vi "CreateArrFileName.vi"(4 "BaseDataPath":path, 6 "VarParName":string, 7 "Date":string, 8 "error in (no error)":errorcluster, 9 "PointIndex":i64, 10 "ScanIndex":i64, 11 "SessionInd":i32) -> (0 "error out":errorcluster, 1 "DataFileName":path, 2 "HeadersFileName":path)   [LabVIEW 2019, in "Interface.lvclass"]
doc: "Ce VI sauvegarde les données d'acquisition pour en garder une copie de sécurité qui peut être rappeller en cas de panne."
uses:
  Interface Class/Interface.lvclass
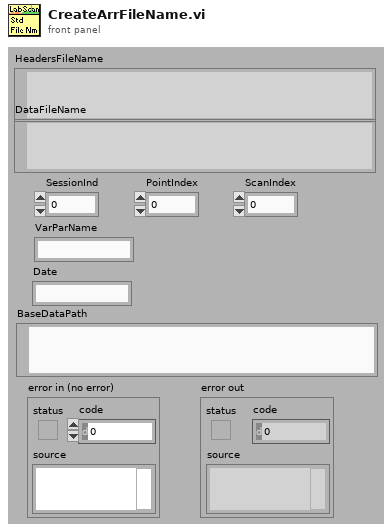
[diagram p1: front panel]
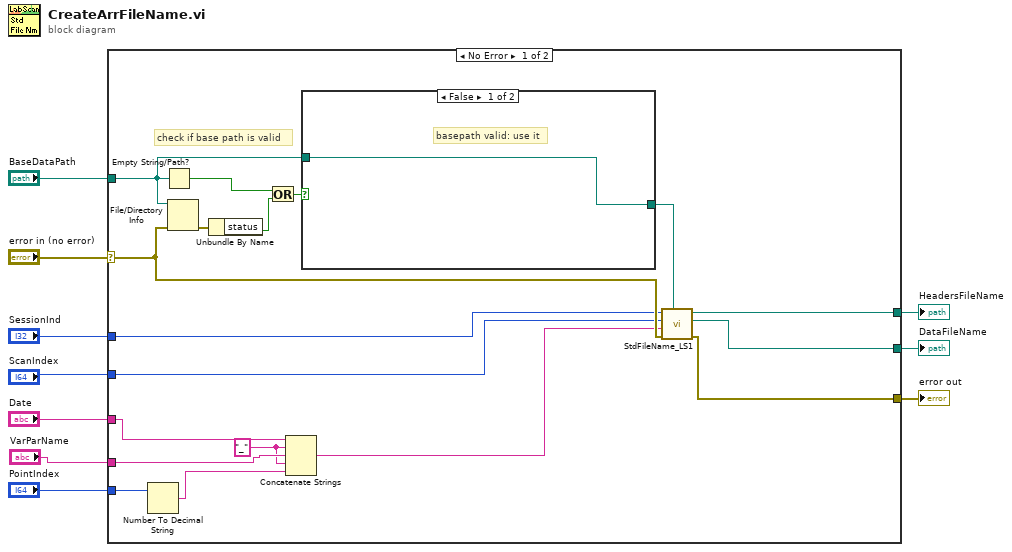
[diagram p0: block diagram]
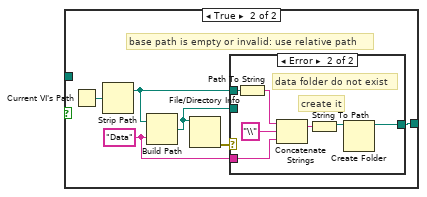
[diagram p2: hidden frame]
diagram:
  n1 = case shown="No Error" "error in (no error)" {
    selector: "error in (no error)" -> [w22 w44]
    tunnel: [w24 w44] -> w9
    tunnel: "Date" -> [w16 _]
    tunnel: [w21 _] -> w7
    tunnel: [w20 _] -> w6
    tunnel: "ScanIndex" -> [w19 _]
    tunnel: "BaseDataPath" -> [w18 _]
    tunnel: "SessionInd" -> [w17 _]
    tunnel: "VarParName" -> [w15 _]
    tunnel: "PointIndex" -> [w13 _]
    frame No Error {
      w14 = "_" ("chaîne")
      # "check if base path is valid"
      n2 = Number To Decimal String(number=w13) -> (decimal integer string=w12:string)  [unwired: 1 in]
      n3 = Empty String/Path?(string/path=w18) -> (empty?=w28:bool)
      n4 = File/Directory Info(path=w18, error in=w22) -> (error out=w27:errorcluster)  [unwired: 6 out]
      n5 = Unbundle By Name(w27) -> ("status"=w26:bool)
      n6 = Or(x=w28, y=w26) -> (x .or. y?=w25:bool)
      n7 = Concatenate Strings(w16, w14, w15, w14, w12) -> (w11:string)
      n8 = case shown="False" w25 {
        tunnel: [w29 w34] -> w23
        tunnel: w18 -> [w29 _]
        frame False {
          # "basepath valid: use it"
        }
        frame True {
          w32 = "Data" ("nom ou chemin relatif")
          # "base path is empty or invalid: use relative path"
          n9 = Current VI's Path() -> (path=w35:path)
          n10 = Strip Path(path=w35) -> (stripped path=w33:path)  [unwired: 1 out]
          n11 = Build Path(base path=w33, name or relative path=w32) -> (appended path=w30:path)
          n12 = File/Directory Info(path=w30) -> (error out=w31:errorcluster)  [unwired: 1 in, 6 out]
          n13 = case shown="Error" w31 {
            tunnel: [w36 w43] -> w34
            tunnel: w33 -> [_ w42]
            tunnel: w32 -> [_ w38]
            tunnel: w30 -> [w36 _]
            frame No Error {
            }
            frame Error {
              # "create it"
              # "data folder do not exist"
              n14 = Path To String(path=w42) -> (string=w41:string)
              n15 = Concatenate Strings(w41, "\\" ("chaîne"), w38) -> (w40:string)
              n16 = String To Path(string=w40) -> (path=w39:path)
              n17 = Create Folder(path (use dialog)=w39) -> (created path=w43:path)  [unwired: 2 in, 2 out]
            }
          }
        }
      }
      n18 = call "StdFileName_LS1.vi"("chemin de base"=w23, "error in (no error)"=w22, "Date"=w11, "Scan"=w19, "Session"=w17) -> ("error out"=w24:errorcluster, "chemin Data"=w21:path, "chemin Headers"=w20:path)  [unwired: 2 in, 2 out]
    }
    frame Error {
    }
  }
  "error out" <- w9
  "DataFileName" <- w7
  "HeadersFileName" <- w6
